vi "Water Level Test.vi"() -> ()   [LabVIEW 2012]
uses:
  <vilib>/ActorFramework/Actor/Actor.lvclass
  <vilib>/ActorFramework/Stop Msg/Stop Msg.lvclass
  Water Level/Water Level.lvclass
  Level Controller/Level Controller/Level Controller.lvclass
  <vilib>/ActorFramework/Message Queue/Message Queue.lvclass
panel:
  in  "stop":bool
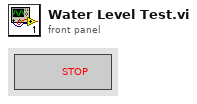
[diagram p1: front panel]
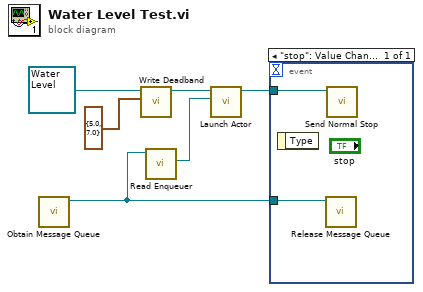
[diagram p0: block diagram]
diagram:
  n1 = call <vilib>:"Obtain Message Queue.vi"() -> ("Message Queue"=w6:refnum<class "Message Queue.lvclass">)  [unwired: 10 in, 1 out]
  n2 = call "Write Deadband.vi"("Deadband"=cluster{"LO":dbl, "HI":dbl} {"LO"=5.0, "HI"=7.0}, "Level Controller in"=refnum<class "Water Level.lvclass"> refnum ("Water Level.lvclass")) -> ("Level Controller out"=w2:refnum<class "Level Controller.lvclass">)  [unwired: 8 in, 1 out]
  n3 = call <vilib>:"Read Enqueuer.vi"("Message Queue"=w6) -> ("Message Enqueuer"=w4:refnum<class "Message Enqueuer.lvclass">)  [unwired: 10 in]
  n4 = call <vilib>:"Launch Actor.vi"("Actor-to-Caller Enqueuer"=w4, "Actor"=w2) -> ("Caller-To-Actor Enqueuer"=w5:refnum<class "Message Enqueuer.lvclass">)  [unwired: 8 in, 1 out]
  n5 = event shown="[0] \"stop\": Value Change" {
    selector: _ -> [_]
    dyn-events: _ -> [_]
    timeout: _ -> [_]
    tunnel: w5 -> [w8]
    tunnel: w6 -> [w7]
    event "stop": Value Change {
      n6 = event-data() -> ()  [unwired: 1 in, 1 out]
      n7 = call <vilib>:"Release Message Queue.vi"("Message Queue"=w7) -> ()  [unwired: 9 in, 2 out]
      n8 = call <vilib>:"Send Normal Stop.vi"("Message Enqueuer"=w8) -> ()  [unwired: 10 in, 1 out]
    }
  }
